vi "CUST Get PDC Real Data.vi"(10 "pseudoPdcId":i32, 11 "rd":T1) -> (2 "function return":i32, 3 "rd out":T1)   [LabVIEW 2013, in "C37118-DLL.lvlib"]
doc: "STRONGRIDIEEEC37118DLL_API int __cdecl getPdcRealData(pdcDataFrame* rd, int32_t pseudoPdcId);"
uses:
  C37118-DLL.lvlib
  builds/StrongridDLL/StrongridDLL.dll
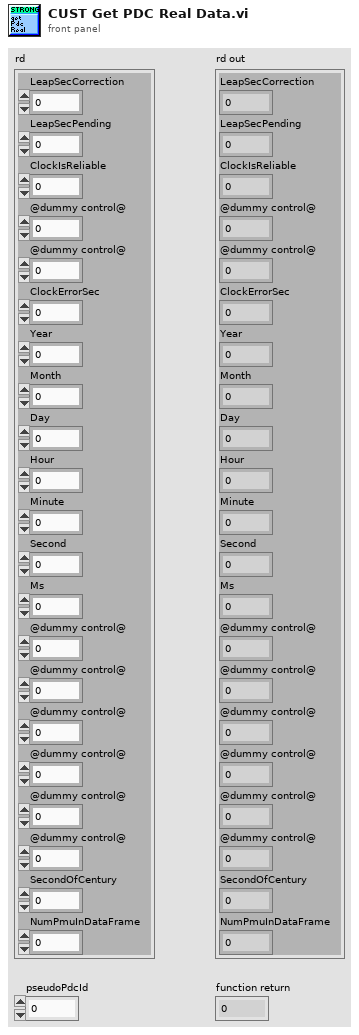
[diagram p1: front panel]
types:
  T1 = cluster{"LeapSecCorrection":i32, "LeapSecPending":u8, "ClockIsReliable":u8, "@dummy control@":i8, "@dummy control@":i8, "ClockErrorSec":sgl, "Year":i16, "Month":i16, "Day":i16, "Hour":i16, "Minute":i16, "Second":i16, "Ms":i16, "@dummy control@":i8, "@dummy control@":i8, "@dummy control@":i8, "@dummy control@":i8, "@dummy control@":i8, "@dummy control@":i8, "SecondOfCentury":dbl, "NumPmuInDataFrame":i32}
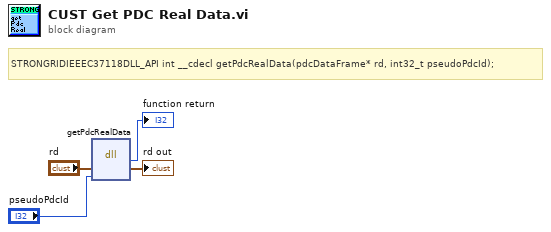
[diagram p0: block diagram]
diagram:
  # "STRONGRIDIEEEC37118DLL_API int __cdecl getPdcRealData(pdcDataFrame* rd, int32_t pseudoPdcId);"
  n1 = dll-call lib="C:/dev/OSS/S3DK/builds/StrongridDLL/StrongridDLL.*" fn="getPdcRealData"("rd"="rd", "pseudoPdcId"="pseudoPdcId") -> (→"function return":i32, "rd"=→"rd out":T1)  [unwired: 4 in, 2 out]
